vi "GPU_Process.vi"(8 "DataFlag":i32=1, 9 "Ann Array Params":T5={"Synth Foc?"=FALSE, "Focal Zones"=41, "Switch T/R"=0, "Trans Geometry (mm)"={"Transducer"=0, "Geo Focus"=12.0, "a (radius)"=3.0, "# of rings"=5, "kerf space "=0.1, "Center Freq"=12.0}, "Sub Ap Excite?"=FALSE, "Full Array Scan?"=FALSE, "Xmt/Rcv"={"XMIT"=[TRUE, TRUE, TRUE, TRUE, TRUE], "RCV"=[TRUE, TRUE, TRUE, TRUE, TRUE]}, "PulseSpacing (us)"=0.0, "Xmit Ring"=0, "XMIT CHS"=0, "RCV CHS"=0, "GPU?"=FALSE, "Save TIFF?"=FALSE, "downfactor"=1, "RCV 1CH"=0} {"RCV 1CH" items=["All", "1", "2", "3", "4", "5"]; "Trans Geometry (mm)"."Transducer" items=["6D 12R 40 MHz"=0, "10D 31R 20 MHz"=1, "10D 23R 20 MHz"=2, "6D 23R 40 MHz"=3, "4.5D 10.7R 40 MHz"=4, "9D 23.5R 20 MHz"=5, "9D 25.8R 20MHz"=6, "Enter"=99]; "Switch T/R" min=1 max=5 step=1}, 10 "Digitizer Settings":T1 {"Trigger Settings"."Trig Slope" items=["Positive", "Negative"]; "Trigger Settings"."Level (mV)" format="%.2f"; "Trigger Settings"."Trig Coupling" items=["DC 1 MOhm", "AC 1 MOhm", "DC 50 Ohm", "AC 50 Ohm"]; "Trigger Settings"."Trig Source" items=["Chan 1", "External"]; "Rel Dig Delay" format="%.2f"; "DigTimeOut" format="%.2f"; "Avg Num" min=1; "Offset delay (us)" format="%.2f"; "Additional dig delay (us)" format="%.2f"; "Digitizer delay (us)" format="%.2f"}, 11 "Raw Data In":i16[](array[numeric])) -> (0 "nError":i32, 1 "RFimageData":i16[][](array[numeric]), 2 "RF_Out":i16[][](array[numeric]))   [LabVIEW 2022 SP3]
uses:
  Annular Array/-AnnularRoutines/AnnularArray.ctl
  Annular Array/-AnnularRoutines/TransGeometry.ctl
  Annular Array/-AnnularRoutines/ArrayGeometry.ctl
  ScanningControl/Digitizers/-DigitizerRoutines/DigitizerSettings.ctl
  ScanningControl/Digitizers/-DigitizerRoutines/Digitizer.ctl
  ScanningControl/Digitizers/-DigitizerRoutines/DigConfig.ctl
  ScanningControl/Digitizers/-DigitizerRoutines/DigitizerID.ctl
  C:/Windows/System32/ADQAPI_dotNet_helper.dll
  Windows/System32/ADQAPI_dotNet_helper.dll
  ScanningControl/Motion Controllers/-MotionRoutines/MotionGlobals.vi
  GPU_HK/LabVIEW Example/riversideSAFilter-X64.dll
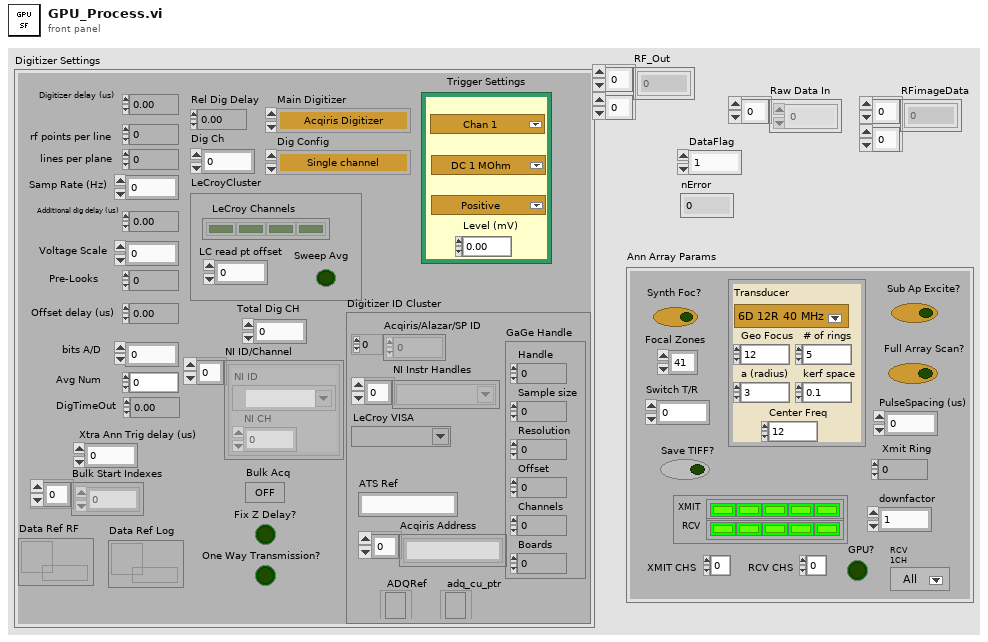
[diagram p1: front panel]
types:
  T1 = typedef "DigitizerSettings.ctl" = cluster{"Digitizer delay (us) ":dbl, "rf points per line":i32, "lines per plane":i32, "Samp Rate (Hz)":dbl, "Additional dig delay (us)":dbl, "Voltage Scale":dbl, "Pre-Looks":i32, "Offset delay (us)":dbl, "bits A/D":i8, "Avg Num":i32, "DigTimeOut":sgl, "Rel Dig Delay":sgl, "Dig Ch":i32, "LeCroyCluster":cluster{"LeCroy Channels":bool[], "LC read pt offset":dbl, "Sweep Avg":bool}, "Main Digitizer":T2, "Dig Config":T3, "Digitizer ID Cluster":T4, "Trigger Settings":cluster{"Trig Source":u16, "Trig Coupling":u16, "Trig Slope":u16, "Level (mV)":dbl}, "Bulk Acq":bool, "Bulk Start Indexes":i32[], "Data Ref RF":refnum<data-value>, "NI ID/Channel":cluster{"NI ID":refnum<k15>, "NI CH":i32}[], "Total Dig CH":i32, "Xtra Ann Trig delay (us)":dbl, "Fix Z Delay?":bool, "One Way Transmission?":bool, "Data Ref Log":refnum<data-value>}
  T2 = typedef "Digitizer.ctl" = enum16{"Acqiris Digitizer", "NI Digitizer", "LeCroy", "GaGe", "AlazarTech", "No Digitizer", "Teledyne"}
  T3 = typedef "DigConfig.ctl" = enum16{"Single channel", "2 Chans w/ 2 Acqiris", "2 Chans w/ 1 Acqiris", "5-CH Pulser New", "5-CH pulser w/ ann array", "5-pass style ann array", "Empty"}
  T4 = typedef "DigitizerID.ctl" = cluster{"Acqiris/Alazar/SP ID":u32[], "NI Instr Handles":refnum<k15>[], "LeCroy VISA":refnum<visa-resource-name>, "GaGe Handle":cluster{"Handle":u32, "Sample size":u32, "Resolution":i32, "Offset":i32, "Channels":u32, "Boards":u32}, "ATS Ref":string, "Acqiris Address":string[], "ADQRef":refnum<k24>, "adq_cu_ptr":refnum<k24>}
  T5 = typedef "AnnularArray.ctl" = cluster{"Synth Foc?":bool, "Focal Zones":i16, "Switch T/R":i16, "Trans Geometry (mm)":T6, "Sub Ap Excite?":bool, "Full Array Scan?":bool, "Xmt/Rcv":cluster{"XMIT":bool[], "RCV":bool[]}, "PulseSpacing (us)":sgl, "Xmit Ring":i32, "XMIT CHS":u8, "RCV CHS":u8, "GPU?":bool, "Save TIFF?":bool, "downfactor":i32, "RCV 1CH":u16}
  T6 = typedef "TransGeometry.ctl" = cluster{"Transducer":T7, "Geo Focus":dbl, "a (radius)":dbl, "# of rings":i32, "kerf space ":dbl, "Center Freq":dbl}
  T7 = typedef "ArrayGeometry.ctl" = u16
  T8 = cluster{"low cutoff":i32, "order":i32, "high cutoff":i32}
  T9 = cluster{"txPos":i32[], "rxPos":i32[], "Weights":i16[], "Ones":i16[]}
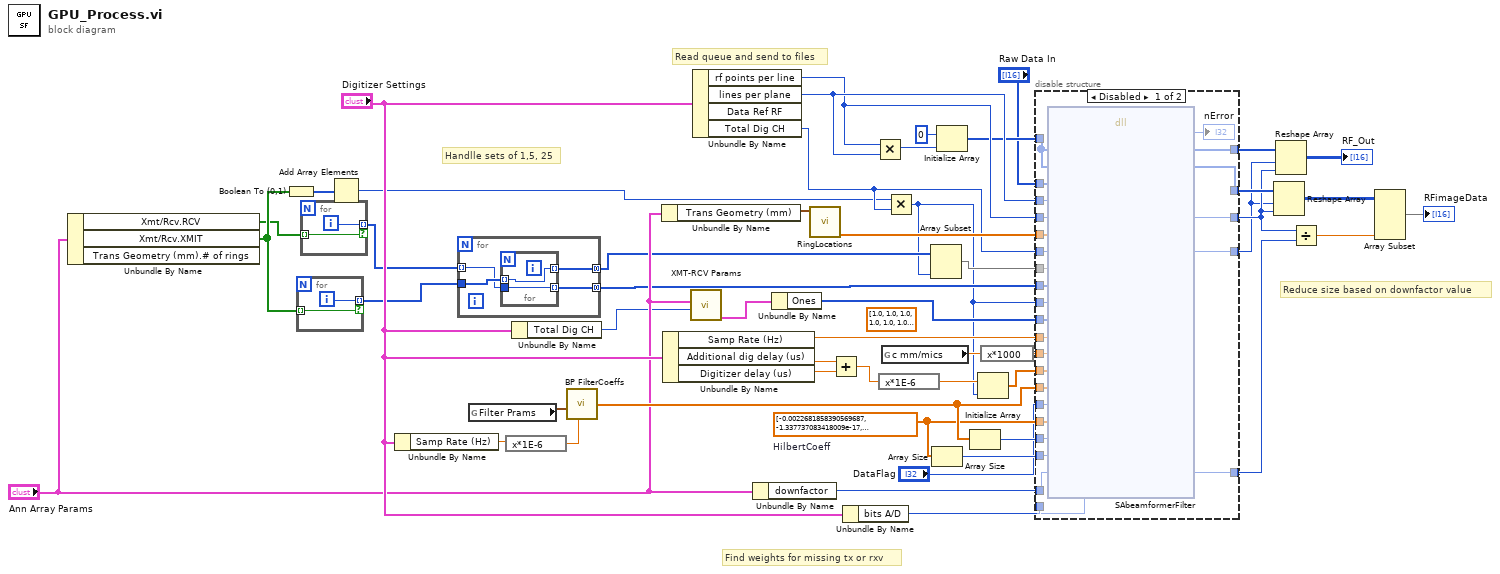
[diagram p0: block diagram]
diagram:
  (unwired) sgl[] [1.0, 1.0, 1.0, 1.0, 1.0, 1.0, 1.0, 1.0, 1.0, 1.0, 1.0, 1.0, 1.0, 1.0, 1.0, 1.0, 1.0, 1.0, 1.0, 1.0, 1.0, 1.0, 1.0, 1.0, 1.0, 1.0, 1.0, 1.0, 1.0, 1.0, 1.0, 1.0, 1.0, 1.0, 1.0, 1.0, 1.0, 1.0, 1.0, 1.0, 1.0, 1.0, 1.0, 1.0, 1.0, 1.0, 1.0, 1.0, 1.0, 1.0] ("weighting")
  w47 = sgl[] [-0.0022681858, -1.3377371e-17, -0.0041749156, 1.3026156e-17, -0.0068346895, -4.195826e-17, -0.010427003, -1.1244341e-16, -0.015182828, -3.725316e-17, -0.021423787, -1.1259981e-16, -0.029640518, -9.678795e-17, -0.040659484, -5.638797e-17, -0.05603469, 9.1425055e-18, -0.079112425, -9.958648e-17, -0.118650794, 1.000237e-18, -0.20691232, -6.3757414e-17, -0.6348398, 0.0, 0.6348398, 6.3757414e-17, 0.20691232, -1.000237e-18, 0.118650794, 9.958648e-17, 0.079112425, -9.1425055e-18, 0.05603469, 5.638797e-17, 0.040659484, 9.678795e-17, 0.029640518, 1.1259981e-16, 0.021423787, 3.725316e-17, 0.015182828, 1.1244341e-16, 0.010427003, 4.195826e-17, 0.0068346895, -1.3026156e-17, 0.0041749156, 1.3377371e-17, 0.0022681858]  # HilbertCoeff
  # "Find weights for missing tx or rxv"
  # "Reduce size based on downfactor value"
  # "Handlle sets of 1,5, 25"
  # "Read queue and send to files"
  n1 = Unbundle By Name("Ann Array Params") -> ("Xmt/Rcv.RCV"=w5:bool[], "Xmt/Rcv.XMIT"=w8:bool[])  [unwired: 1 out]
  n2 = Boolean To (0,1)(Boolean=w8) -> (0, 1=w9:i16[])
  n3 = for {
    tunnel: w8 -> [w52] mode=indexing
    tunnel: [w53] -> w6 mode=indexing if=w52
    i -> [w53]
  }
  n4 = for {
    tunnel: w5 -> [w54] mode=indexing
    tunnel: [w55] -> w4 mode=indexing if=w54
    i -> [w55]
  }
  n5 = Add Array Elements(numeric array=w9) -> (sum=w7:i16)
  n6 = Unbundle By Name("Digitizer Settings") -> ("Samp Rate (Hz)"=w30:dbl)
  n7 = for {
    tunnel: [w59] -> w3 mode=concatenating
    tunnel: [w58] -> w10 mode=concatenating
    tunnel: w6 -> [w57]
    tunnel: w4 -> [w56] mode=indexing
    n8 = for {
      tunnel: [w60] -> w59 mode=indexing
      tunnel: w56 -> [w61]
      tunnel: [w61] -> w58 mode=indexing
      tunnel: w57 -> [w60] mode=indexing
    }
  }
  n9 = global read "MotionGlobals.vi" "Filter Prams"() -> (w29:T8)
  n10 = expression code="x*1E-6"(w30) -> (w28:dbl)
  n11 = Unbundle By Name("Digitizer Settings") -> ("Total Dig CH"=w13:i32)
  n12 = call "BP FilterCoeffs.vi"("sample rate MHz"=w28, "Filter Prams"=w29) -> ("FIR Windowed Coefficients"=w49:dbl[])  [unwired: 4 in]
  n13 = Unbundle By Name("Ann Array Params") -> ("Trans Geometry (mm)"=w43:T6)
  n14 = Unbundle By Name("Digitizer Settings") -> ("Samp Rate (Hz)"=w36:dbl, "Additional dig delay (us)"=w39:dbl, "Digitizer delay (us)"=w40:dbl)
  n15 = call "XMT-RCV Params.vi"("Dig Channels"=w13, "Ann Array Params"="Ann Array Params") -> ("GPU ordering"=w12:T9)  [unwired: 4 in, 5 out]
  n16 = Unbundle By Name("Digitizer Settings") -> ("rf points per line"=w44:i32, "lines per plane"=w45:i32, "Total Dig CH"=w15:i32)  [unwired: 1 out]
  n17 = Unbundle By Name("Ann Array Params") -> ("downfactor"=w51:i32)
  n18 = Unbundle By Name(w12) -> ("Ones"=w11:i16[])
  n19 = call "RingLocations.vi"("Trans Geometry (mm)"=w43) -> ("GPU Geometry"=w32:dbl[])  [unwired: 9 in, 1 out]
  n20 = Add(x=w39, y=w40) -> (x+y=w41:dbl)
  n21 = Unbundle By Name("Digitizer Settings") -> ("bits A/D"=w16:i8)
  n22 = Multiply(x=w44, y=w45) -> (x*y=w34:i32)
  n23 = expression code="x*1E-6"(w41) -> (w46:dbl)
  n24 = global read "MotionGlobals.vi" "c mm/mics"() -> (w37:sgl)
  n25 = Multiply(x=w7, y=w15) -> (x*y=w1:i32)
  n26 = Array Subset(array=w3, length=w1) -> (w2:i32[])  [unwired: 1 in]
  n27 = Array Size(array=w47) -> (size(s)=w48:i32)
  n28 = Initialize Array(i16 0 ("element"), w34) -> (w35:i16[])
  n29 = Array Size(array=w49) -> (size(s)=w50:i32)
  n30 = Initialize Array(w46, w1) -> (w42:dbl[])
  n31 = expression code="x*1000"(w37) -> (w38:sgl)
  n32 = disable-structure shown="Disabled" {
    disable-tunnel: w51 -> [w87 _]
    disable-tunnel: w50 -> [w86 _]
    disable-tunnel: w49 -> [w85 _]
    disable-tunnel: w48 -> [w84 _]
    disable-tunnel: w47 -> [w83 _]
    disable-tunnel: w45 -> [w82 _]
    disable-tunnel: w44 -> [w81 _]
    disable-tunnel: w42 -> [w80 _]
    disable-tunnel: w38 -> [w79 _]
    disable-tunnel: w36 -> [w78 _]
    disable-tunnel: w35 -> [w77 _]
    disable-tunnel: w32 -> [w76 _]
    disable-tunnel: "Raw Data In" -> [w75 _]
    disable-tunnel: "DataFlag" -> [w74 _]
    disable-tunnel: [w72 _] -> w26
    disable-tunnel: [w71 _] -> w25
    disable-tunnel: [w70 _] -> w23
    disable-tunnel: [w69 _] -> w22
    disable-tunnel: [w68 _] -> w21
    disable-tunnel: w16 -> [w67 _]
    disable-tunnel: w15 -> [w66 _]
    disable-tunnel: w11 -> [w65 _]
    disable-tunnel: w10 -> [w64 _]
    disable-tunnel: w2 -> [w63 _]
    disable-tunnel: w1 -> [w62 _]
    frame Disabled {
      n33 = dll-call lib="D:/LabVIEWSuite_64_OS/GPU_HK/LabVIEW Example/riversideSAFilter-X64.dll" fn="SAbeamformerFilter"("RF_Out"=w77, "RFimage"=w77, "RFdata"=w75, "numScanline"=w82, "dataVectorLength"=w81, "TdrGeometry"=w76, "numChannel"=w66, "txPos"=w63, "rxPos"=w64, "numTxRxPair"=w62, "weighting"=w65, "fs"=w78, "sos"=w79, "time_start"=w80, "BPfilter"=w85, "DataFlag"=w74, "filter"=w83, "BPFILTERLENGTH"=w86, "FILTERLENGTH"=w84, "downfactor"=w87, "ADbits"=w67) -> ("nError"=→"nError":i32, "RF_Out"=w71:i16[], "RFimage"=w70:i16[], "numScanline"=w68:i32, "dataVectorLength"=w69:i32, "downfactor"=w72:i32)  [unwired: 19 in, 2 out]
    }
    frame Enabled {
    }
  }
  n34 = Reshape Array(w23, w21, w22) -> (w20:i16[][])
  n35 = Reshape Array(w25, w21, w22) -> (→"RF_Out":i16[][])
  n36 = Divide(x=w22, y=w26) -> (x/y=w18:dbl)
  n37 = Array Subset(array=w20, length (col)=w18) -> (→"RFimageData":i16[][])  [unwired: 3 in]
